vi "Image Global Variable.vi"() -> ()   [LabVIEW 2013]
panel:
  out "sCMOS Image":u16[][](graph)
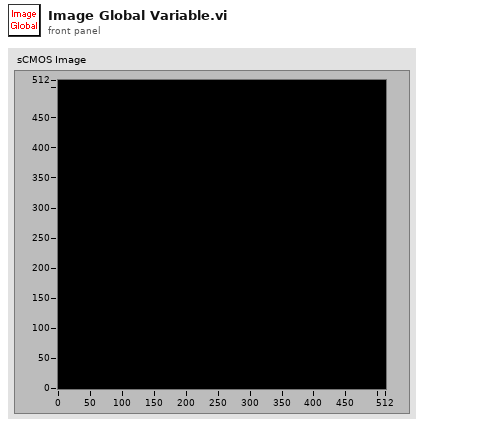
[diagram p1: front panel]
diagram:
